vi "Start.vi"(8 "error in (no error)":errorcluster, 11 "App Watcher in":refnum<class "App Watcher.lvclass">) -> (0 "error out":errorcluster, 3 "App Watcher out":refnum<class "App Watcher.lvclass">)   [LabVIEW 2020, in "PicoG-App.lvlib" / "App Watcher.lvclass"]
uses:
  App Watcher.lvclass
  Watcher Loop Async.vi
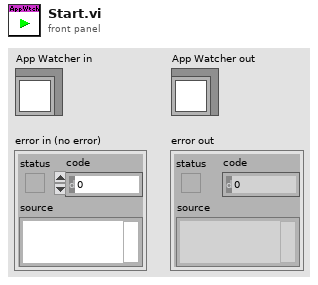
[diagram p1: front panel]
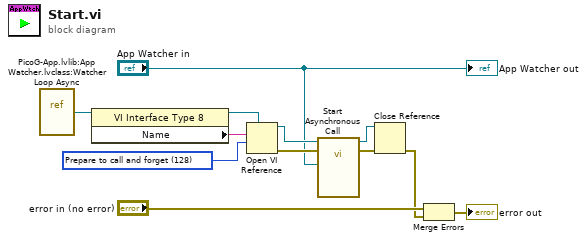
[diagram p0: block diagram]
diagram:
  w6 = 128 items=["Record modifications"=1, "Open templates for editing"=2, "Prompt user to save"=4, "Prepare for reentrant run"=8, "Prompt to find missing subVIs"=16, "Hide loading dialog box"=32, "Enable simultaneous calls"=64, "Prepare to call and forget"=128, "Simultaneous call and forget"=192, "Prepare to call and collect"=256, "Simultaneous call and collect"=320]
  n1 = vi-ref "PicoG-App.lvlib:App Watcher.lvclass:Watcher Loop Async.vi"() -> (w4:refnum<vi>)
  n2 = property class="VI Interface Type 8"(reference=w4) -> (reference out=w7:refnum<vi>, "Name"=w5:string)  [unwired: 1 in, 1 out]
  n3 = Open VI Reference(type specifier VI Refnum (for type only)=w7, vi path=w5, options=w6) -> (vi reference=w9:refnum<vi>, error out=w8:errorcluster)  [unwired: 3 in]
  n4 = call-by-ref "Start Asynchronous Call"(reference=w9, error in=w8, "App Watcher in"="App Watcher in") -> (reference out=w11:refnum<vi>, error out=w10:errorcluster)  [unwired: 11 in]
  n5 = Close Reference(reference=w11, error in (no error)=w10) -> (error out=w1:errorcluster)
  n6 = Merge Errors("error in (no error)", w1) -> (→"error out":errorcluster)
  "App Watcher out" <- "App Watcher in"
